vi "Get State.vi"(8 "error in (no error)":errorcluster, 11 "Command in":refnum<class "Command Actor.lvclass">) -> (0 "error out":errorcluster, 1 "Command State String":string, 3 "Command out":refnum<class "Command Actor.lvclass">)   [LabVIEW 2014, in "Robot Actor Framework.lvlib" / "Command Actor.lvlib" / "Command Actor.lvclass"]
uses:
  Command Actor.lvclass
  Command Actor.lvclass/Command Actor.ctl
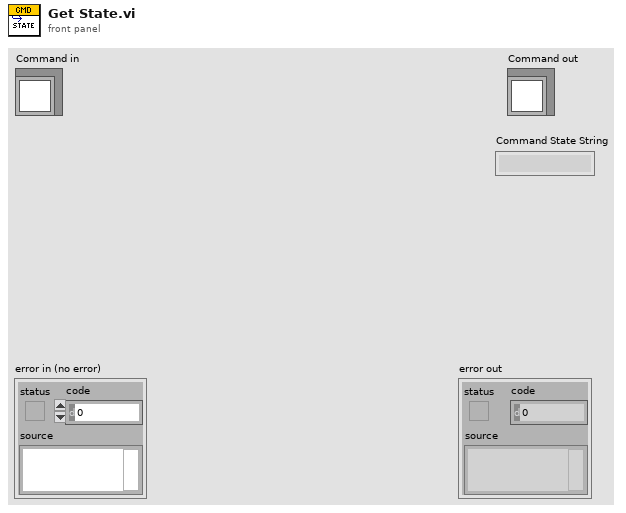
[diagram p1: front panel]
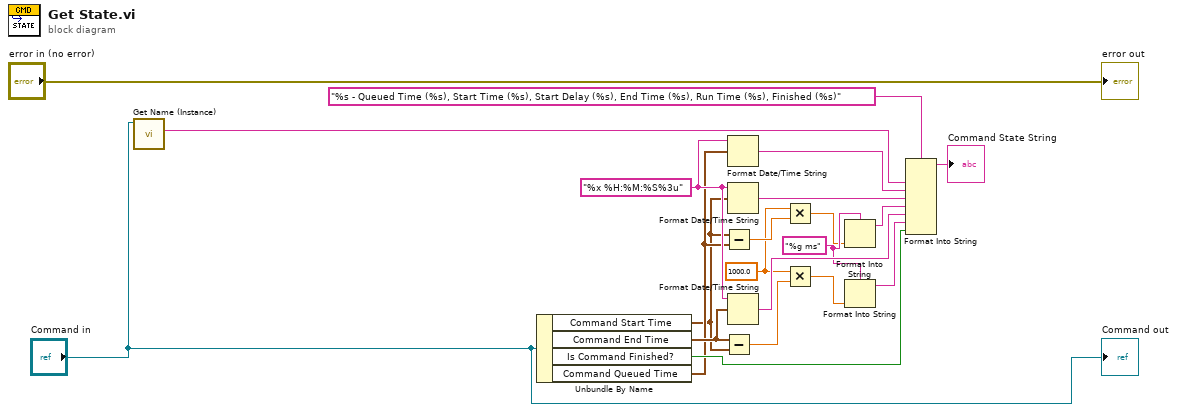
[diagram p0: block diagram]
diagram:
  w1 = 1000.0 ("x")
  w9 = "%g ms" ("format string")
  w16 = "%x %H:%M:%S%3u" ("time format string (%c)")
  n1 = call-dynamic "Get Name (Instance).vi"("Command Actor in"="Command in") -> ("Name (Instance)"=w17:string)  [unwired: 8 in, 2 out]
  n2 = Unbundle By Name("Command in") -> ("Command Start Time"=w4:timestamp, "Command End Time"=w12:timestamp, "Is Command Finished?"=w11:bool, "Command Queued Time"=w5:timestamp)
  n3 = Subtract(x=w4, y=w5) -> (x-y=w8:dbl)
  n4 = Subtract(x=w12, y=w4) -> (x-y=w7:dbl)
  n5 = Format Date/Time String(time format string (%c)=w16, seconds (now)=w5) -> (date/time string=w15:string)  [unwired: 1 in]
  n6 = Format Date/Time String(time format string (%c)=w16, seconds (now)=w4) -> (date/time string=w14:string)  [unwired: 1 in]
  n7 = Format Date/Time String(time format string (%c)=w16, seconds (now)=w12) -> (date/time string=w13:string)  [unwired: 1 in]
  n8 = Multiply(x=w1, y=w8) -> (x*y=w2:dbl)
  n9 = Multiply(x=w1, y=w7) -> (x*y=w3:dbl)
  n10 = Format Into String(format string=w9, w2) -> (resulting string=w10:string)  [unwired: 2 in, 1 out]
  n11 = Format Into String(format string=w9, w3) -> (resulting string=w6:string)  [unwired: 2 in, 1 out]
  n12 = Format Into String(format string="%s - Queued Time (%s), Start Time (%s), Start Delay (%s), End Time (%s), Run Time (%s), Finished (%s)", w17, w15, w14, w10, w13, w6, w11) -> (resulting string=→"Command State String":string)  [unwired: 2 in, 1 out]
  "error out" <- "error in (no error)"
  "Command out" <- "Command in"
